vi "Construct Initial Filter Sequence.vi"(8 "error in":errorcluster, 11 "Seq Builder in":refnum<class "Cal Sequence Builder.lvclass">) -> (0 "error out":errorcluster, 2 "Init Filter":refnum<class "STEP.lvclass">[](array[class]), 3 "Seq Builder out":refnum<class "Cal Sequence Builder.lvclass">)   [LabVIEW 2015, in "Cal Sequence Builder.lvclass"]
uses:
  Cal Sequence Builder.lvclass
  Reusable/Sequence/STEPS/STEP.lvclass
  Change Filter State/Change Filter Position.lvclass
  Wait/Wait.lvclass
  Wait/Wait.lvclass/Wait.ctl
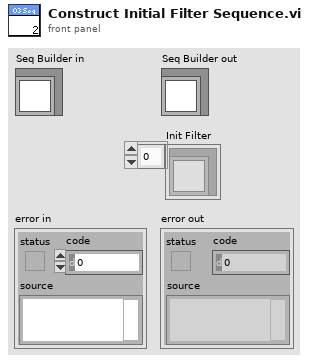
[diagram p1: front panel]
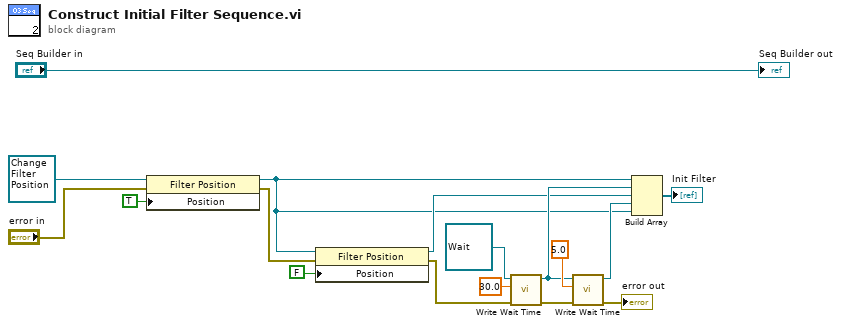
[diagram p0: block diagram]
diagram:
  n1 = property class="Filter Position"(reference=refnum<class "Change Filter Position.lvclass"> refnum ("Filter Position"), error in="error in", "Position"=TRUE) -> (reference out=w3:refnum<class "Change Filter Position.lvclass">, error out=w7:errorcluster)
  n2 = property class="Filter Position"(reference=w3, error in=w7, "Position"=FALSE) -> (reference out=w10:refnum<class "Change Filter Position.lvclass">, error out=w6:errorcluster)
  n3 = call "Write Wait Time.vi"("error in (no error)"=w6, "Wait Time"=30.0, "Wait in"=refnum<class "Wait.lvclass"> refnum ("Wait")) -> ("error out"=w5:errorcluster, "Wait out"=w11:refnum<class "Wait.lvclass">)  [unwired: 7 in]
  n4 = call "Write Wait Time.vi"("error in (no error)"=w5, "Wait Time"=5.0, "Wait in"=w11) -> ("error out"=→"error out":errorcluster, "Wait out"=w9:refnum<class "Wait.lvclass">)  [unwired: 7 in]
  n5 = Build Array(w3, w11, w10, w9, w3) -> (→"Init Filter":refnum<class "STEP.lvclass">[])
  "Seq Builder out" <- "Seq Builder in"
